vi "DATE-DT Byte Stream to Timestamp.vi"(8 "error in (no error)":errorcluster, 10 "Byte Stream":u8[](array[numeric])) -> (0 "error out":errorcluster, 2 "Value":timestamp)   [LabVIEW 2018, in "TwinCAT ADS.lvclass"]
uses:
  TwinCAT ADS.lvclass
  TwinCAT.Ads
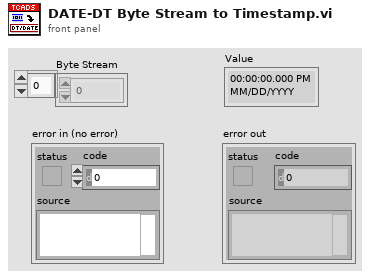
[diagram p1: front panel]
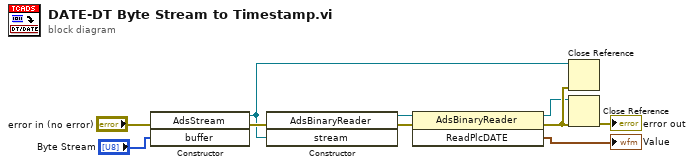
[diagram p0: block diagram]
diagram:
  n1 = constructor class="AdsStream"(error in="error in (no error)", "buffer"="Byte Stream") -> (reference out=w7:refnum<k24>, error out=w8:errorcluster)  [unwired: 2 in, 2 out]
  n2 = constructor class="AdsBinaryReader"(error in=w8, "stream"=w7) -> (reference out=w10:refnum<k24>, error out=w9:errorcluster)  [unwired: 2 in, 2 out]
  n3 = invoke class="AdsBinaryReader" method="ReadPlcDATE"(reference=w10, error in=w9) -> (reference out=w5:refnum<k24>, error out=w6:errorcluster, "ReadPlcDATE"=→"Value":timestamp)  [unwired: 1 in]
  n4 = Close Reference(reference=w7, error in (no error)=w6) -> ()  [unwired: 1 out]
  n5 = Close Reference(reference=w5, error in (no error)=w6) -> (error out=→"error out":errorcluster)
